vi "Read Delta T.vi"(8 "error in (no error)":errorcluster, 11 "3010 in":refnum<class "3010.lvclass">) -> (0 "error out":errorcluster, 2 "dT":dbl, 3 "3010 out":refnum<class "3010.lvclass">)   [LabVIEW 2014, in "3010.lvclass"]
uses:
  3010.lvclass
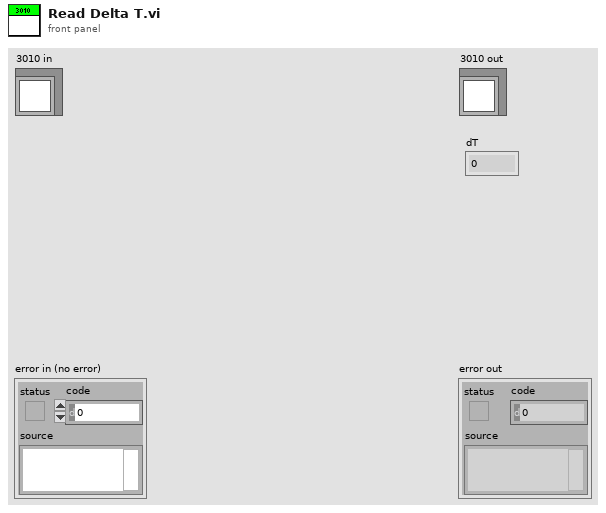
[diagram p1: front panel]
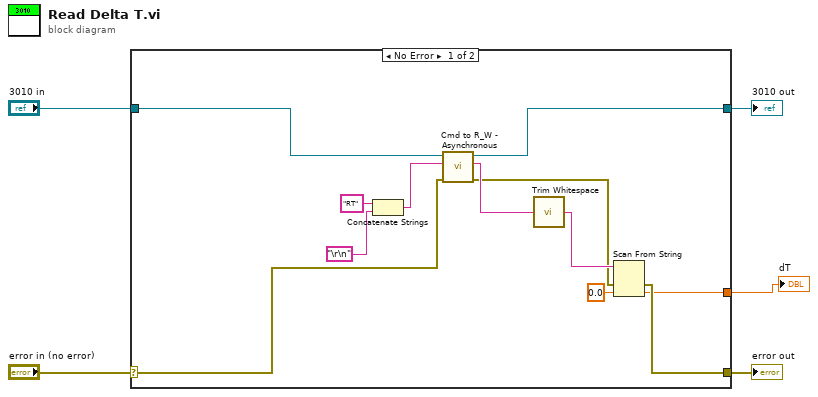
[diagram p0: block diagram]
diagram:
  n1 = case shown="No Error" "error in (no error)" {
    selector: "error in (no error)" -> [w8 w19]
    tunnel: [w7 w19] -> w4
    tunnel: [w9 w18] -> w2
    tunnel: "3010 in" -> [w10 w18]
    tunnel: [w6 _] -> w1
    frame No Error {
      n2 = Concatenate Strings("RT" ("string"), "\r\n") -> (w15:string)
      n3 = call-dynamic "Cmd to R_W - Asynchronous.vi"("error in"=w8, "write buffer"=w15, "Serial IO in"=w10) -> ("error out"=w11:errorcluster, "read buffer"=w14:string, "Serial IO out"=w9:refnum<class "3010.lvclass">)  [unwired: 6 in]
      n4 = call <vilib>:"Trim Whitespace.vi"("string"=w14) -> ("trimmed string"=w13:string)  [unwired: 1 in]
      n5 = Scan From String(input string=w13, error in=w11, default 1=0.0 ("default value 1")) -> (error out=w7:errorcluster, output 1=w6:dbl)  [unwired: 2 in, 2 out]
    }
    frame Error {
    }
  }
  "error out" <- w4
  "3010 out" <- w2
  "dT" <- w1
